vi "controlGroundTargetRange.vi"(7 "Set":bool, 8 "error in":errorcluster, 9 "GroundTargetRange":i32, 10 "axis in":u8, 11 "connection ID":refnum<k5>) -> (0 "error out":errorcluster, 1 "GroundTargetRange out":i32, 2 "axis out":i32, 3 "connection ID":refnum<k5>)   [LabVIEW 2015, in "AMC_VIs.lvlib"]
doc: "Retrieves or sets the range around the target position in which the auto grounding becomes active."
uses:
  AMC_VIs.lvlib
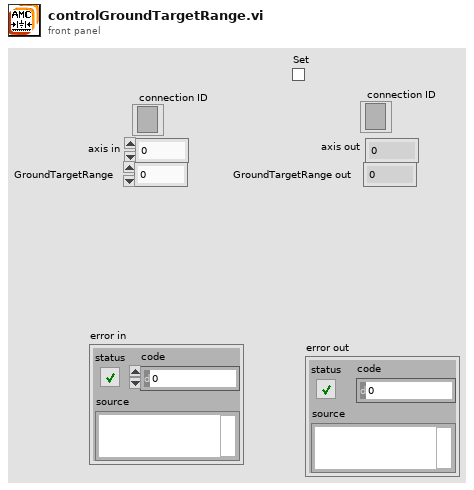
[diagram p1: front panel]
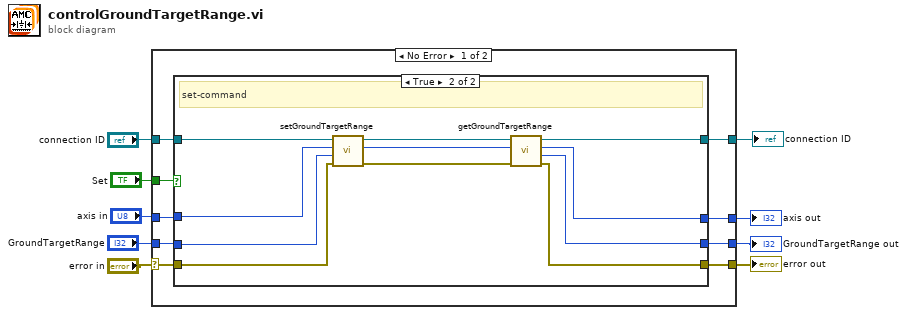
[diagram p0: block diagram]
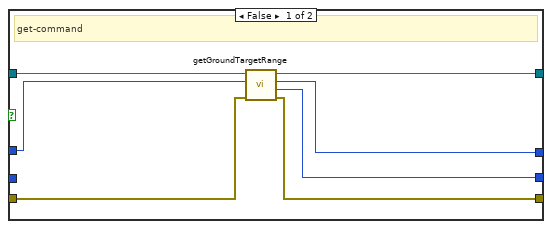
[diagram p2: hidden frame]
diagram:
  n1 = case shown="No Error" "error in" {
    selector: "error in" -> [w14 w40]
    tunnel: "axis in" -> [w18 w37]
    tunnel: [w10 w40] -> w8
    tunnel: "GroundTargetRange" -> [w16 w38]
    tunnel: [w13 w38] -> w3
    tunnel: "Set" -> [w15 _]
    tunnel: [w12 w39] -> w6
    tunnel: "connection ID" -> [w17 w39]
    tunnel: [w11 w37] -> w1
    frame No Error {
      n2 = case shown="True" w15 {
        tunnel: w17 -> [w21 w36]
        tunnel: w18 -> [w22 w33]
        tunnel: w16 -> [_ w32]
        tunnel: w14 -> [w25 w31]
        tunnel: [w23 w27] -> w13
        tunnel: [w20 w34] -> w12
        tunnel: [w19 w28] -> w11
        tunnel: [w24 w26] -> w10
        frame False {
          # "get-command"
          n3 = call "getGroundTargetRange.vi"("error in"=w25, "axis"=w22, "connection ID"=w21) -> ("error out"=w24:errorcluster, "targetrange"=w23:i32, "axis_out"=w19:i32, "connection ID"=w20:refnum<k5>)  [unwired: 5 in]
        }
        frame True {
          # "set-command"
          n4 = call "setGroundTargetRange.vi"("error in"=w31, "range"=w32, "axis"=w33, "connection ID"=w36) -> ("error out"=w30:errorcluster, "axis_out"=w29:i32, "connection ID"=w35:refnum<k5>)  [unwired: 5 in]
          n5 = call "getGroundTargetRange.vi"("error in"=w30, "axis"=w29, "connection ID"=w35) -> ("error out"=w26:errorcluster, "targetrange"=w27:i32, "axis_out"=w28:i32, "connection ID"=w34:refnum<k5>)  [unwired: 5 in]
        }
      }
    }
    frame Error {
    }
  }
  "error out" <- w8
  "axis out" <- w1
  "GroundTargetRange out" <- w3
  "connection ID" <- w6
